vi "CustomAPDSpectrum.vi"(0 "LightField Automation":refnum<class "LightField Automation.lvclass">, 1 "PH_Init_Data":T2, 3 "PH_Settings_Params":T1={"SyncDiv"=1, "DeviceIndex"=0, "CFD0 level"=50, "CFD0 zero X"=10, "CFD1 level"=50, "CFD1 zero X"=10, "Range No."=0, "StopOnOverflow"=FALSE, "AcqTime (ms)"=0.0} {"Range No." min=0 max=5 step=1; "CFD1 zero X" min=0 max=40 step=1; "CFD1 level" min=0 max=400 step=1; "CFD0 zero X" min=-1300 max=400 step=10; "CFD0 level" min=-1300 max=400 step=10; "SyncDiv" min=1 max=8 step=1}, 4 "Stop Spectrum Custom":refnum<vi>, 5 "HR mode":u16(ring)=3 caption="Which HR?" items=["Excitation"=1, "Detection"=2], 7 "LightField Automation error":errorcluster, 9 "Center Wavelength (nm)":refnum<vi>, 11 "Center2 Wavelength (nm)":refnum<vi>, 12 "Scan Spectrum Progess Bar":refnum<vi>, 13 "CCD 1D Spectrum Main 3":refnum<vi>, 14 "Mono2 Wavelength (nm)":refnum<vi>, 16 "Scan Spectrum Cust Exp Params 2":T3) -> (15 "WLs":dbl[](array[numeric]), 17 "PL2":dbl[][](array[numeric]), 20 "LFA Out":refnum<class "LightField Automation.lvclass">, 25 "PL":dbl[](array[numeric]), 27 "LFA Error Out":errorcluster)   [LabVIEW 2019]
uses:
  C:/Users/manip/Documents/Controle_Manip_2020/Thorlabs.MotionControl.KCube.SolenoidCLI.dll
  Thorlabs.MotionControl.KCube.SolenoidCLI.dll
  Light Field/lightfield-automation-labview/LightField Automation.lvclass
panel:
  out "CCD 1D Spectrum Main 2":cluster{dbl[], dbl[]}[](graph) caption="Main spectrum"
  in  "Mono2 Wavelength (nm)":dbl=300.0 caption="Wavelength (nm)" min=300.0 max=1000.0 step=0.1
  out "CustCase":bool
  in  "ESP300 COM Port":refnum<visa-resource-name>="COM4" caption="COM Port"
  in  "Scan Spectrum Progess Bar":u8(slide) scale=0.0..100.0
  in  "Stop Spectrum Custom 2":bool
  in  "Stop Spectrum Custom":bool
  out "Acq Time (ms)":dbl
  out "NumPoints":dbl
  out "KCube Shutter On?":bool
  out "Spectrum Custom Mode":u16
  out "Spectrum End Wavelength (nm)":dbl
  out "Spectrum Step Wavelength (nm)":dbl
  out "Spectrum Start Wavelength (nm)":dbl
  in  "Photodiode error out":errorcluster caption="error out" {"code" format="%.0x"}
  in  "Scan Spectrum Cust Exp Params":T4
  in  "Photodiode handle out":refnum<visa-resource-name> caption="instrument handle out"
  in  "Center Wavelength (nm)":dbl=490.12 caption="Center WL :"
  out "Excitation Power (uW)":dbl=0.2 caption="P    =" format="%#_3p"
  out "CCD 1D Spectrum Main":cluster{dbl[], dbl[]}(graph)
  out "Shutter Ctrls":u16(ring)
  out "KCube Shutter Device Reference":refnum<k24>
types:
  T1 = cluster{"SyncDiv":i32, "DeviceIndex":i32, "CFD0 level":i32, "CFD0 zero X":i32, "CFD1 level":i32, "CFD1 zero X":i32, "Range No.":i32, "StopOnOverflow":bool, "AcqTime (ms)":dbl}
  T2 = cluster{"Deviceindex":i32, "Initialization Status":string, "DLL Version":string, "Initialization Error":bool, "Status":string, "Calib Error":bool}
  T3 = cluster{"Acq Time (ms)":dbl, "Spectrum Start Wavelength (nm)":dbl, "Spectrum Step Wavelength (nm)":dbl, "Spectrum End Wavelength (nm)":dbl, "Spectrum Custom Mode":u16, "KCube Shutter On?":bool}
  T4 = cluster{"Spectrum Start Wavelength (nm)":dbl, "Spectrum Step Wavelength (nm)":dbl, "Spectrum End Wavelength (nm)":dbl, "Spectrum Custom Mode":u16, "KCube Shutter On?":bool}
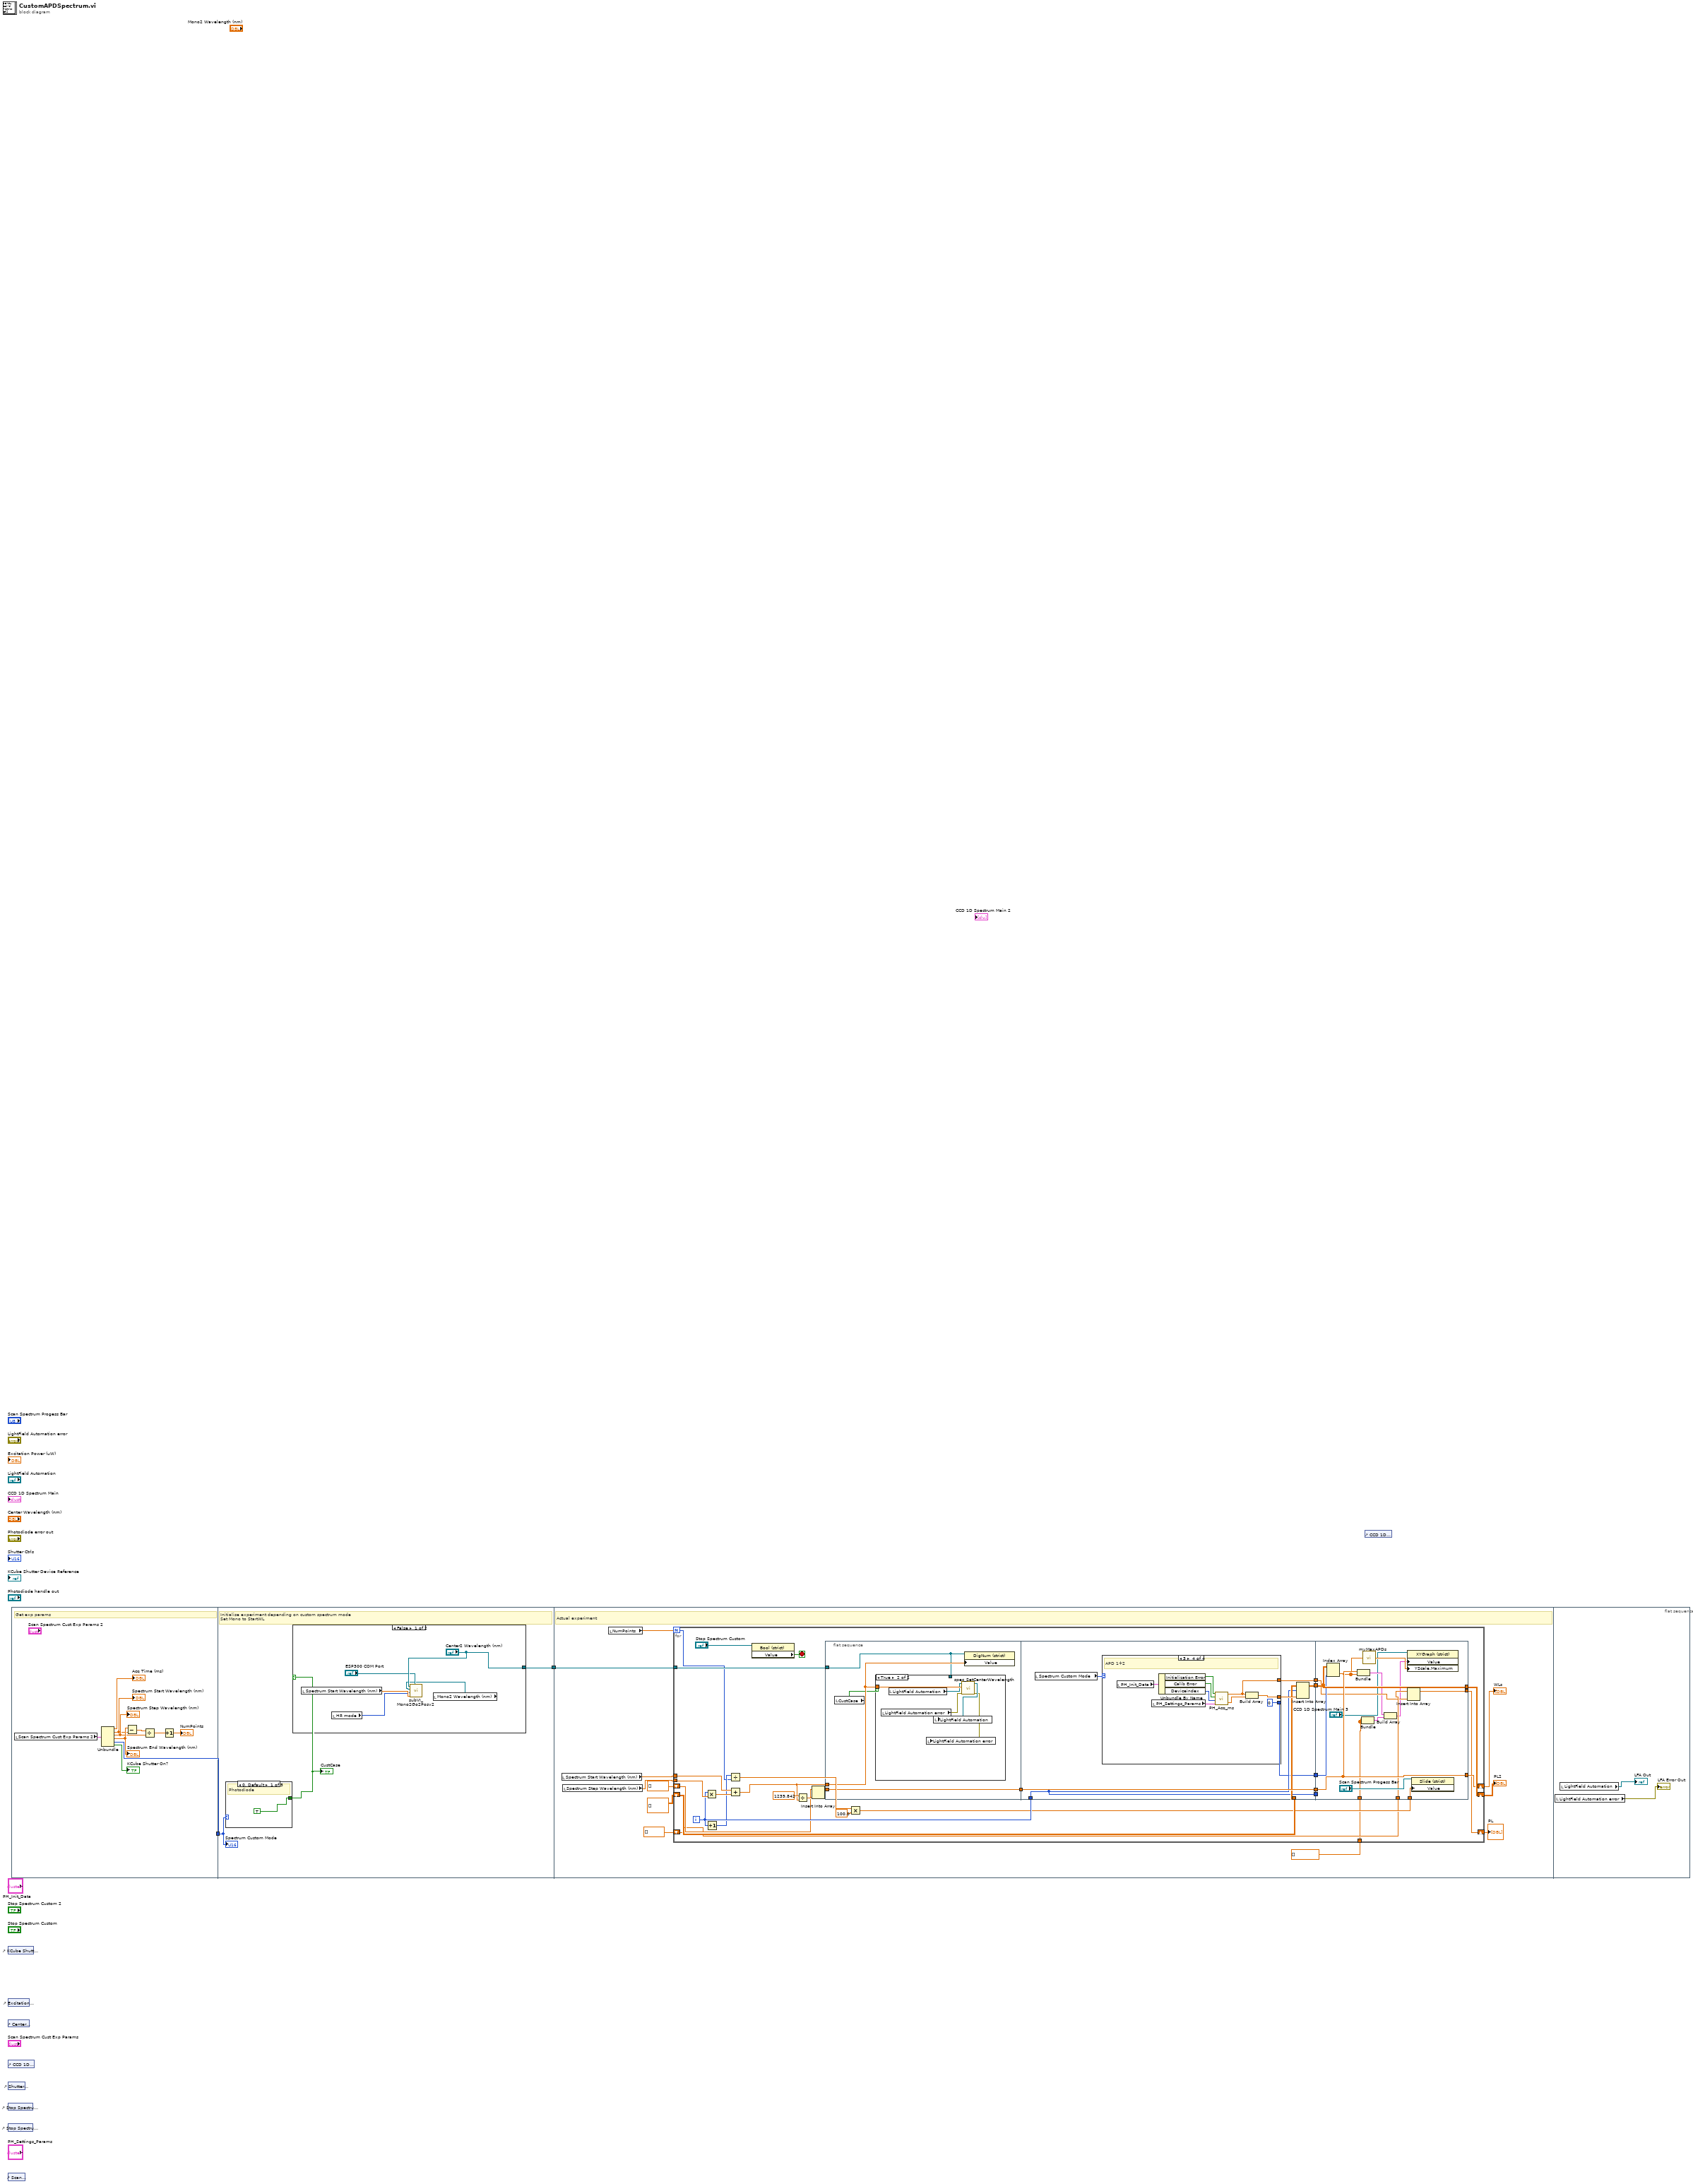
[diagram p0: block diagram]
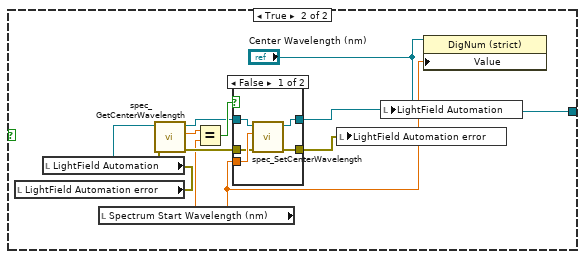
[diagram p2: hidden frame]
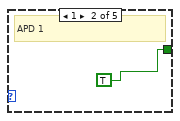
[diagram p4: hidden frame]
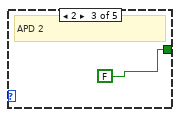
[diagram p5: hidden frame]
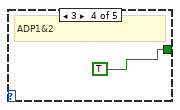
[diagram p6: hidden frame]
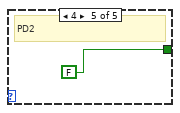
[diagram p7: hidden frame]
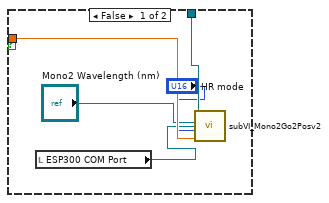
[diagram p8: hidden frame]
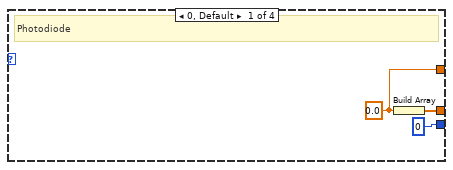
[diagram p9: hidden frame]
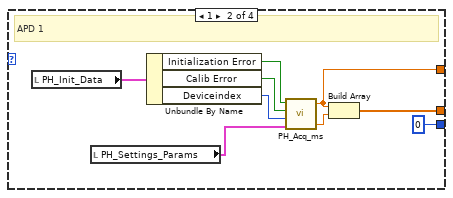
[diagram p10: hidden frame]
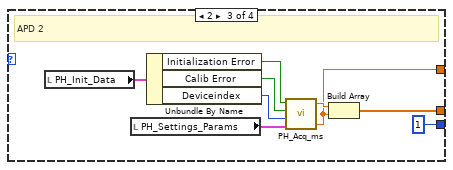
[diagram p11: hidden frame]
diagram:
  n1 = control-ref of="KCube Shutter Device Reference"() -> ()  [unwired: 1 out]
  n2 = control-ref of="Excitation Power (uW)"() -> ()  [unwired: 1 out]
  n3 = control-ref of="Center Wavelength (nm)"() -> ()  [unwired: 1 out]
  n4 = control-ref of="CCD 1D Spectrum Main"() -> ()  [unwired: 1 out]
  n5 = control-ref of="Shutter Ctrls"() -> ()  [unwired: 1 out]
  n6 = control-ref of="Stop Spectrum Custom"() -> ()  [unwired: 1 out]
  n7 = control-ref of="Stop Spectrum Custom 2"() -> ()  [unwired: 1 out]
  n8 = control-ref of="Scan Spectrum Progess Bar"() -> ()  [unwired: 1 out]
  n9 = flat-sequence {
    tunnel: [w7] -> w2
    tunnel: w2 -> [w15]
    tunnel: [w14] -> w1
    tunnel: w1 -> [w50]
    frame #0 {
      # "Get exp params"
      n10 = local read "Scan Spectrum Cust Exp Params 2"() -> (w12:T3)
      n11 = Unbundle(w12) -> ("Acq Time (ms)"=→"Acq Time (ms)":dbl, "Spectrum Start Wavelength (nm)"=w4:dbl, "Spectrum Step Wavelength (nm)"=w5:dbl, "Spectrum End Wavelength (nm)"=w6:dbl, "Spectrum Custom Mode"=w7:u16, "KCube Shutter On?"=→"KCube Shutter On?":bool)
      "Spectrum Start Wavelength (nm)" <- w4
      "Spectrum Step Wavelength (nm)" <- w5
      "Spectrum End Wavelength (nm)" <- w6
      n12 = Subtract(x=w6, y=w4) -> (x-y=w11:dbl)
      n13 = Divide(x=w11, y=w5) -> (x/y=w10:dbl)
      n14 = Increment(x=w10) -> (x+1=→"NumPoints":dbl)
    }
    frame #1 {
      # "Initialise experiment depending on custom spectrum mode\nSet Mono to StartWL"
      n15 = case shown="0, Default" w15 {
        tunnel: [TRUE TRUE FALSE TRUE FALSE] -> w13
        frame 0, Default {
          # "Photodiode"
        }
        frame 1 {
          # "APD 1"
        }
        frame 2 {
          # "APD 2"
        }
        frame 3 {
          # "ADP1&2"
        }
        frame 4 {
          # "PD2"
        }
      }
      "CustCase" <- w13
      n16 = case shown="False" w13 {
        tunnel: ["Center2 Wavelength (nm)" "Center Wavelength (nm)"] -> w14
        frame False {
          n17 = local read "Spectrum Start Wavelength (nm)"() -> (w18:dbl)
          n18 = local read "HR mode"() -> (w17:u16)
          n19 = local read "Mono2 Wavelength (nm)"() -> (w16:refnum<vi>)
          n20 = call "subVI_Mono2Go2Posv2.vi"("Mono2 Motor Pos"="Center2 Wavelength (nm)", "Mono2 Wavelength (nm)"=w16, "HR mode"=w17, "Postion (Unit)"=w18, "ESP300 COM Port"="ESP300 COM Port") -> ()  [unwired: 2 out]
        }
        frame True {
          n21 = local read "LightField Automation error"() -> (w22:errorcluster)
          n22 = local read "LightField Automation"() -> (w21:refnum<class "LightField Automation.lvclass">)
          n23 = local read "Spectrum Start Wavelength (nm)"() -> (w26:dbl)
          n24 = call "spec_GetCenterWavelength.vi"("error in (no error)"=w22, "LightField Automation in"=w21) -> ("error out"=w27:errorcluster, "Center Wavelength"=w30:dbl, "LightField Automation out"=w28:refnum<class "LightField Automation.lvclass">)  [unwired: 7 in]
          n25 = Equal?(x=w30, y=w26) -> (x = y?=w29:bool)
          n26 = case shown="False" w29 {
            tunnel: w28 -> [w33 w37]
            tunnel: w27 -> [w34 w36]
            tunnel: [w32 w37] -> w25
            tunnel: [w31 w36] -> w24
            tunnel: w26 -> [w35 _]
            frame False {
              n27 = call "spec_SetCenterWavelength.vi"("error in (no error)"=w34, "Center Wavelength"=w35, "LightField Automation in"=w33) -> ("error out"=w31:errorcluster, "LightField Automation out"=w32:refnum<class "LightField Automation.lvclass">)  [unwired: 7 in]
            }
            frame True {
            }
          }
          n28 = local write "LightField Automation error"(w24) -> ()
          n29 = local write "LightField Automation"(w25) -> ()
          n30 = property class="DigNum (strict)"(reference="Center Wavelength (nm)", "Value"=w26) -> ()  [unwired: 1 in, 2 out]
        }
      }
      "Spectrum Custom Mode" <- w15
    }
    frame #2 {
      # "Actual experiment"
      n31 = local read "Spectrum Start Wavelength (nm)"() -> (w52:dbl)
      n32 = local read "Spectrum Step Wavelength (nm)"() -> (w53:dbl)
      n33 = local read "NumPoints"() -> (w51:dbl)
      n34 = for {
        N: w51 -> [w67]
        tunnel: w53 -> [w81]
        tunnel: w52 -> [w80]
        tunnel: w50 -> [w79]
        shift-right: [w72] -> w47
        shift-left: dbl[] [] -> [w58]
        shift-right: [w73] -> w46
        shift-left: dbl[][] [] -> [w74]
        shift-right: [w56] -> w44
        shift-left: dbl[] [] -> [w57]
        tunnel: dbl[] [] -> [w54]
        i -> [w69]
        stop <- w70 stop-if-true
        n35 = Multiply(x=w69, y=w81) -> (x*y=w82:dbl)
        n36 = Increment(x=w69) -> (x+1=w68:i32)
        n37 = Divide(x=w68, y=w67) -> (x/y=w66:dbl)
        n38 = Add(x=w80, y=w82) -> (x+y=w62:dbl)
        n39 = property class="Bool (strict)"(reference="Stop Spectrum Custom") -> ("Value"=w70:bool)  [unwired: 1 in, 2 out]
        n40 = Divide(x=1239.842, y=w62) -> (x/y=w61:dbl)
        n41 = Insert Into Array(array=w58, new element=w61) -> (w75:dbl[])  [unwired: 1 in]
        n42 = flat-sequence {
          tunnel: [w86] -> w77
          tunnel: w75 -> [w86]
          tunnel: w79 -> [w84]
          tunnel: w62 -> [w85]
          tunnel: w74 -> [w100]
          tunnel: w69 -> [w99]
          tunnel: [w102] -> w78
          tunnel: w77 -> [w101]
          tunnel: [w101] -> w76
          tunnel: [w99] -> w60
          tunnel: [w98] -> w59
          tunnel: [w97] -> w55
          tunnel: w78 -> [w146]
          tunnel: w76 -> [w149]
          tunnel: [w149] -> w72
          tunnel: [w146] -> w73
          tunnel: w64 -> [w147]
          tunnel: w60 -> [_]
          tunnel: w59 -> [w145]
          tunnel: w57 -> [w144]
          tunnel: [w143] -> w56
          tunnel: w55 -> [w142]
          tunnel: w54 -> [w139]
          frame #0 {
            n43 = local read "CustCase"() -> (w83:bool)
            n44 = case shown="True" w83 {
              tunnel: w85 -> [w91 w96]
              tunnel: w84 -> [w89 _]
              frame False {
                n45 = local read "ESP300 COM Port"() -> (w90:refnum<visa-resource-name>)
                n46 = call "subVI_Mono2Go2Posv2.vi"("Mono2 Motor Pos"=w89, "Mono2 Wavelength (nm)"="Mono2 Wavelength (nm)", "HR mode"="HR mode", "Postion (Unit)"=w91, "ESP300 COM Port"=w90) -> ()  [unwired: 2 out]
              }
              frame True {
                n47 = local read "LightField Automation error"() -> (w94:errorcluster)
                n48 = local read "LightField Automation"() -> (w95:refnum<class "LightField Automation.lvclass">)
                n49 = call "spec_SetCenterWavelength.vi"("error in (no error)"=w94, "Center Wavelength"=w96, "LightField Automation in"=w95) -> ("error out"=w92:errorcluster, "LightField Automation out"=w93:refnum<class "LightField Automation.lvclass">)  [unwired: 7 in]
                n50 = local write "LightField Automation error"(w92) -> ()
                n51 = local write "LightField Automation"(w93) -> ()
              }
            }
            n52 = property class="DigNum (strict)"(reference=w84, "Value"=w85) -> ()  [unwired: 1 in, 2 out]
          }
          frame #1 {
            n53 = local read "Spectrum Custom Mode"() -> (w104:u16)
            n54 = case shown="3" w104 {
              tunnel: [w107 w111 w120 w128] -> w103
              tunnel: [0 ("disabled index (col)") 0 ("disabled index (col)") 1 ("disabled index (col)") 0 ("disabled index (col)")] -> w98
              tunnel: [w105 w108 w117 w126] -> w97
              frame 0, Default {
                w105 = 0.0
                # "Photodiode"
                n55 = Build Array(w105) -> (w107:dbl[])
              }
              frame 1 {
                # "APD 1"
                n56 = local read "PH_Init_Data"() -> (w115:T2)
                n57 = local read "PH_Settings_Params"() -> (w116:T1)
                n58 = Unbundle By Name(w115) -> ("Initialization Error"=w114:bool, "Calib Error"=w113:bool, "Deviceindex"=w112:i32)
                n59 = call "PH_Acq_ms.vi"("PH_Settings_Params"=w116, "Deviceindex"=w112, "Calib Error"=w113, "Initialization Error"=w114) -> ("CH1MeanRate"=w110:dbl, "SyncMeanRate"=w108:dbl)  [unwired: 1 out]
                n60 = Build Array(w108, w110) -> (w111:dbl[])
              }
              frame 2 {
                # "APD 2"
                n61 = local read "PH_Init_Data"() -> (w124:T2)
                n62 = local read "PH_Settings_Params"() -> (w125:T1)
                n63 = Unbundle By Name(w124) -> ("Initialization Error"=w123:bool, "Calib Error"=w122:bool, "Deviceindex"=w121:i32)
                n64 = call "PH_Acq_ms.vi"("PH_Settings_Params"=w125, "Deviceindex"=w121, "Calib Error"=w122, "Initialization Error"=w123) -> ("CH1MeanRate"=w117:dbl, "SyncMeanRate"=w118:dbl)  [unwired: 1 out]
                n65 = Build Array(w118, w117) -> (w120:dbl[])
              }
              frame 3 {
                # "APD 1+2"
                n66 = local read "PH_Init_Data"() -> (w133:T2)
                n67 = local read "PH_Settings_Params"() -> (w134:T1)
                n68 = Unbundle By Name(w133) -> ("Initialization Error"=w132:bool, "Calib Error"=w131:bool, "Deviceindex"=w130:i32)
                n69 = call "PH_Acq_ms.vi"("PH_Settings_Params"=w134, "Deviceindex"=w130, "Calib Error"=w131, "Initialization Error"=w132) -> ("CH1MeanRate"=w129:dbl, "SyncMeanRate"=w126:dbl)  [unwired: 1 out]
                n70 = Build Array(w126, w129) -> (w128:dbl[])
              }
            }
            n71 = Insert Into Array(array=w100, index (row)=w99, new element=w103) -> (w102:dbl[][])  [unwired: 1 in]
          }
          frame #2 {
            n72 = Index Array(array=w146, index (col)=w145) -> (element=w141:dbl[])  [unwired: 1 in]
            n73 = Bundle(w149, w141) -> (w137:cluster{dbl[], dbl[]})  [unwired: 1 in]
            n74 = Bundle(w139, w139) -> (w138:cluster{dbl[], dbl[]})  [unwired: 1 in]
            n75 = call "myMaxAPDs.vi"("Array"=w141) -> ("myMax"=w140:dbl)
            n76 = Build Array(w137, w138) -> (w136:cluster{dbl[], dbl[]}[])
            n77 = property class="XYGraph (strict)"(reference="CCD 1D Spectrum Main 3", "Value"=w136, "YScale.Maximum"=w140) -> ()  [unwired: 1 in, 2 out]
            n78 = Insert Into Array(array=w144, new element=w142) -> (w143:dbl[])  [unwired: 1 in]
            n79 = property class="Slide (strict)"(reference="Scan Spectrum Progess Bar", "Value"=w147) -> ()  [unwired: 1 in, 2 out]
          }
        }
        n80 = Multiply(x=w66, y=100.0) -> (x*y=w64:dbl)
      }
      "WLs" <- w47
      "PL2" <- w46
      "PL" <- w44
    }
    frame #3 {
      n81 = local read "LightField Automation error"() -> (→"LFA Error Out":errorcluster)
      n82 = local read "LightField Automation"() -> (→"LFA Out":refnum<class "LightField Automation.lvclass">)
    }
  }
  n83 = control-ref of="CCD 1D Spectrum Main 2"() -> ()  [unwired: 1 out]
